vi "Write Group #.vi"(8 "error in (no error)":errorcluster, 10 "Group #":i32, 11 "Control-Client in":refnum<class "Control-Client.lvclass">) -> (0 "error out":errorcluster, 3 "Control-Client out":refnum<class "Control-Client.lvclass">)   [LabVIEW 2019, in "Control-Client.lvclass"]
uses:
  Control-Client.lvclass
  Control-Client.lvclass/Control-Client.ctl
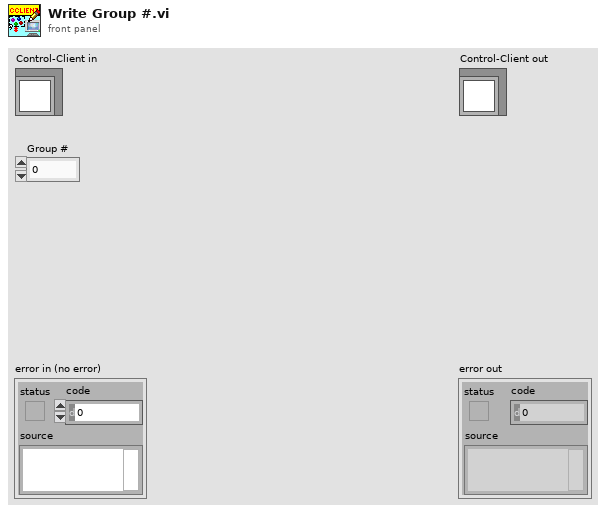
[diagram p1: front panel]
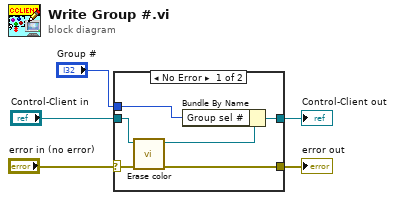
[diagram p0: block diagram]
diagram:
  n1 = case shown="No Error" "error in (no error)" {
    selector: "error in (no error)" -> [w8 w12]
    tunnel: [w7 w12] -> w4
    tunnel: [w11 w13] -> w2
    tunnel: "Control-Client in" -> [w9 w13]
    tunnel: "Group #" -> [w10 _]
    frame No Error {
      n2 = call "Erase color.vi"("error in (no error)"=w8, "Control-Client in"=w9) -> ("error out"=w7:errorcluster, "Control-Client out"=w6:refnum<class "Control-Client.lvclass">)  [unwired: 8 in]
      n3 = Bundle By Name(cluster=w6, "Group sel #"=w10) -> (w11:refnum<class "Control-Client.lvclass">)
    }
    frame Error {
    }
  }
  "error out" <- w4
  "Control-Client out" <- w2
